vi "lvprj2html.vi"() -> ()   [LabVIEW 2014, in "lvprj2html.lvlib"]
uses:
  lvprj2html.lvlib
panel:
  in  "log":string
  in  "inspect dependencies":bool
  in  "generate":bool
  in  "close":bool
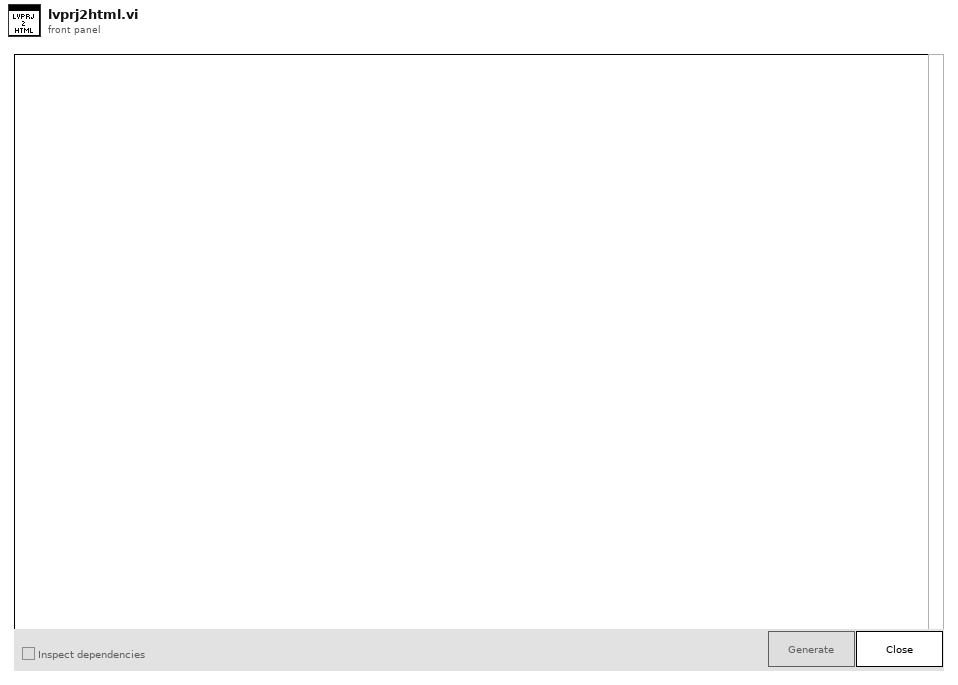
[diagram p1: front panel]
types:
  T1 = enum8{"Enabled", "Disabled", "Disabled and Grayed Out"}
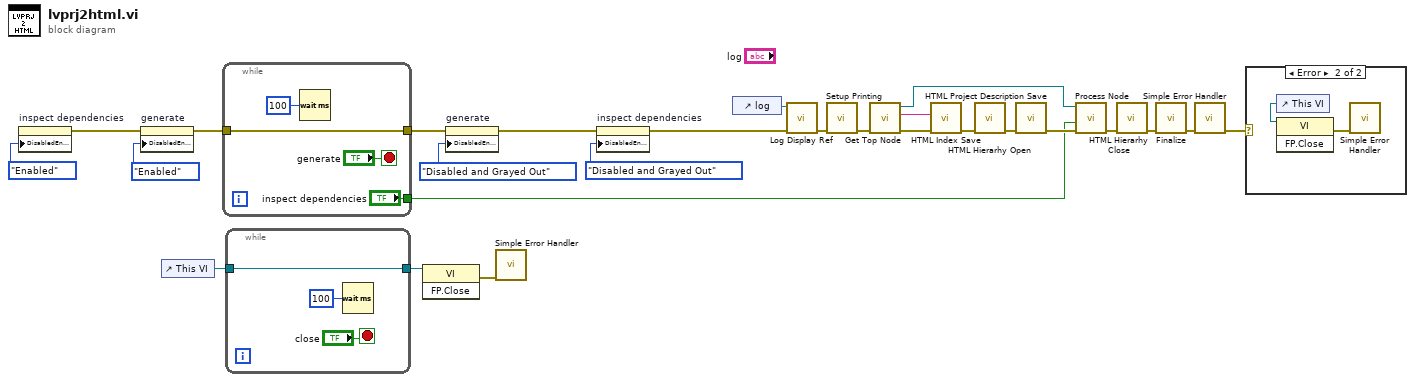
[diagram p0: block diagram]
diagram:
  n1 = property on="inspect dependencies" class="Bool (strict)"("DisabledEnum"=T1."Enabled" ("Disabled")) -> (error out=w5:errorcluster)  [unwired: 2 in, 1 out]
  n2 = property on="generate" class="Bool"(error in=w5, "DisabledEnum"=T1."Enabled" ("Disabled")) -> (error out=w13:errorcluster)  [unwired: 1 in, 1 out]
  n3 = control-ref of="This VI"() -> (w21:refnum<vi>)
  n4 = while {
    tunnel: [w28] -> w18
    tunnel: w13 -> [w28]
    tunnel: ["inspect dependencies"] -> w6
    stop <- "generate" stop-if-true
    n5 = Wait (ms)(milliseconds to wait=u32 100) -> ()  [unwired: 1 out]
  }
  n6 = while {
    tunnel: w21 -> [w31]
    tunnel: [w31] -> w12
    stop <- "close" stop-if-true
    n7 = Wait (ms)(milliseconds to wait=u32 100) -> ()  [unwired: 1 out]
  }
  n8 = invoke class="VI" method="FP.Close"(reference=w12) -> (error out=w11:errorcluster)  [unwired: 2 in, 2 out]
  n9 = property on="generate" class="Bool"(error in=w18, "DisabledEnum"=T1."Disabled and Grayed Out" ("Disabled")) -> (error out=w2:errorcluster)  [unwired: 1 in, 1 out]
  n10 = call <vilib>:"Simple Error Handler.vi"("error in (no error)"=w11) -> ()  [unwired: 4 in, 5 out]
  n11 = property on="inspect dependencies" class="Bool (strict)"(error in=w2, "DisabledEnum"=T1."Disabled and Grayed Out" ("Disabled")) -> (error out=w1:errorcluster)  [unwired: 1 in, 1 out]
  n12 = control-ref of="log"() -> (w22:refnum<vi>)
  n13 = call "Log Display Ref.vi"("error in"=w1, "log display ref"=w22) -> ("error out"=w23:errorcluster)  [unwired: 8 in, 1 out]
  n14 = call "Setup Printing.vi"("error in (no error)"=w23) -> ("error out"=w20:errorcluster)  [unwired: 14 in]
  n15 = call "Get Top Node.vi"("error in (no error)"=w20) -> ("error out"=w9:errorcluster, "top node name"=w7:string, "top node ref"=w26:refnum<vi>)  [unwired: 8 in]
  n16 = call "HTML Index Save.vi"("error in (no error)"=w9, "title"=w7) -> ("error out"=w8:errorcluster)  [unwired: 9 in]
  n17 = call "HTML Hierarhy Open.vi"("error in (no error)"=w8) -> ("error out"=w24:errorcluster)  [unwired: 10 in]
  n18 = call "HTML Project Description Save.vi"("error in (no error)"=w24) -> ("error out"=w19:errorcluster)  [unwired: 10 in]
  n19 = call "Process Node.vi"("error in (no error)"=w19, "inspect dependencies"=w6, "node ref"=w26) -> ("error out"=w25:errorcluster)  [unwired: 8 in]
  n20 = call "HTML Hierarhy Close.vi"("error in"=w25) -> ("error out"=w16:errorcluster)  [unwired: 10 in]
  n21 = call "Finalize.vi"("error in (no error)"=w16) -> ("error out"=w15:errorcluster)  [unwired: 10 in]
  n22 = call <vilib>:"Simple Error Handler.vi"("error in (no error)"=w15) -> ("error out"=w10:errorcluster)  [unwired: 4 in, 4 out]
  n23 = case shown="Error" w10 {
    frame No Error {
    }
    frame Error {
      n24 = control-ref of="This VI"() -> (w34:refnum<vi>)
      n25 = invoke class="VI" method="FP.Close"(reference=w34) -> (error out=w35:errorcluster)  [unwired: 2 in, 2 out]
      n26 = call <vilib>:"Simple Error Handler.vi"("error in (no error)"=w35) -> ()  [unwired: 4 in, 5 out]
    }
  }
